vi "svl_Decimated Exp Avg Level (N Ch).vi"(5 "time constant":dbl=1.0 format="%.3f", 6 "decimation factor":i32=1 min=1 step=1, 7 "exponential mode":enum16{"Slow", "Fast", "Impulse", "Custom"}(ring)=enum."Fast", 8 "error in (no error)":errorcluster, 9 "processing state":T1(ring), 11 "scaled signals":waveform(dbl)[](array[waveform])) -> (0 "error out":errorcluster, 1 "actual time constant [ms]":dbl=125.0 format="%.2f", 3 "scaled signals":waveform(dbl)[](array[waveform]), 4 "actual decimation factor":i32=1 min=1 step=1)   [LabVIEW 2017]
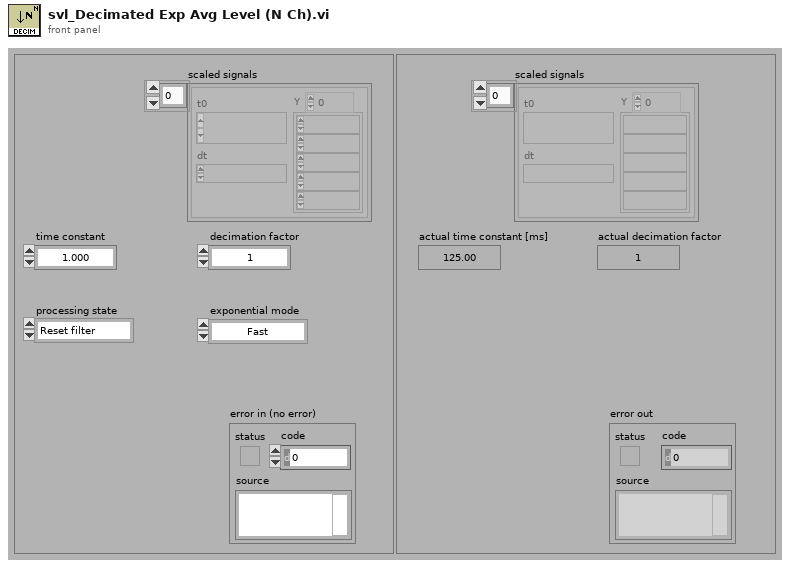
[diagram p1: front panel]
types:
  T1 = enum16{"Reset filter", "Restart averaging", "Continue processing"}
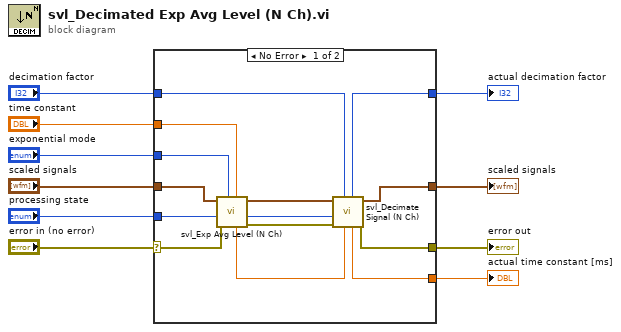
[diagram p0: block diagram]
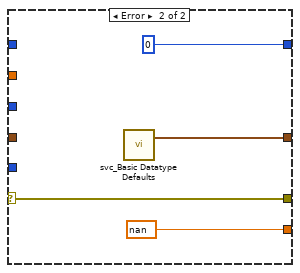
[diagram p2: hidden frame]
diagram:
  n1 = case shown="No Error" "error in (no error)" {
    selector: "error in (no error)" -> [w12 w28]
    tunnel: [w11 w28] -> w10
    tunnel: "exponential mode" -> [w24 _]
    tunnel: [w23 w25] -> w8
    tunnel: "scaled signals" -> [w21 _]
    tunnel: "time constant" -> [w20 _]
    tunnel: "processing state" -> [w19 _]
    tunnel: [w15 nan ("new dt")] -> w4
    tunnel: "decimation factor" -> [w14 _]
    tunnel: [w13 0 ("actual decimation factor")] -> w2
    frame No Error {
      n2 = call <vilib>:"svl_Exp Avg Level (N Ch).vi"("timeConstant"=w20, "exponential mode"=w24, "error in (no error)"=w12, "processing state"=w19, "scaled signals"=w21) -> ("error out"=w18:errorcluster, "dup processing state"=w17:T1, "exp avg signals"=w22:waveform(dbl)[], "actual time constant [ms]"=w16:dbl)  [unwired: 3 in]
      n3 = call <vilib>:"svl_Decimate Signal (N Ch).vi"("actual time constant [ms]"=w16, "decimation factor"=w14, "error in (no error)"=w18, "processing state"=w17, "scaled signals"=w22) -> ("error out"=w11:errorcluster, "decimated signals"=w23:waveform(dbl)[], "dup actual time constant [ms]"=w15:dbl, "actual decimation factor"=w13:i32)  [unwired: 3 in]
    }
    frame Error {
      n4 = call <vilib>:"svc_Basic Datatype Defaults.vi"() -> ("empty array of waveforms"=w25:waveform(dbl)[])  [unwired: 7 in, 12 out]
    }
  }
  "scaled signals" <- w8
  "error out" <- w10
  "actual time constant [ms]" <- w4
  "actual decimation factor" <- w2
